vi "新剖面数据上传.vi"(11 "错误输入（无错误）":errorcluster) -> (15 "error out":errorcluster)   [LabVIEW 2016, in "数据传输系统-03.lvlib"]
uses:
  <vilib>/Utility/config.llb/Write Key (String).vi
  <vilib>/Utility/config.llb/Read Key (String).vi
  <vilib>/Utility/config.llb/NI_LVConfig.lvlib
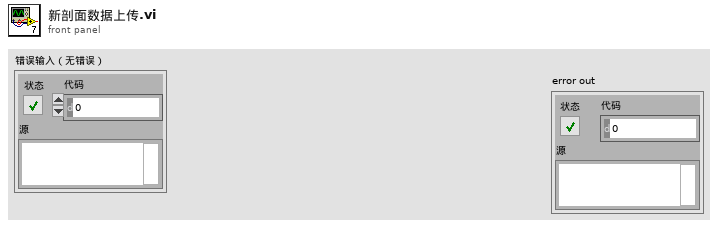
[diagram p1: front panel]
types:
  T1 = cluster{"setini":string, "sysini":string, "hechaini":string, "actualwrite":string, "actualread":string, "datasent":string, "反控命令信息队列":string, "反控与仪器交互":string}
  T2 = typedef "NI_LVConfig.lvlib/Config Data RefNum.ctl" = refnum<k1>
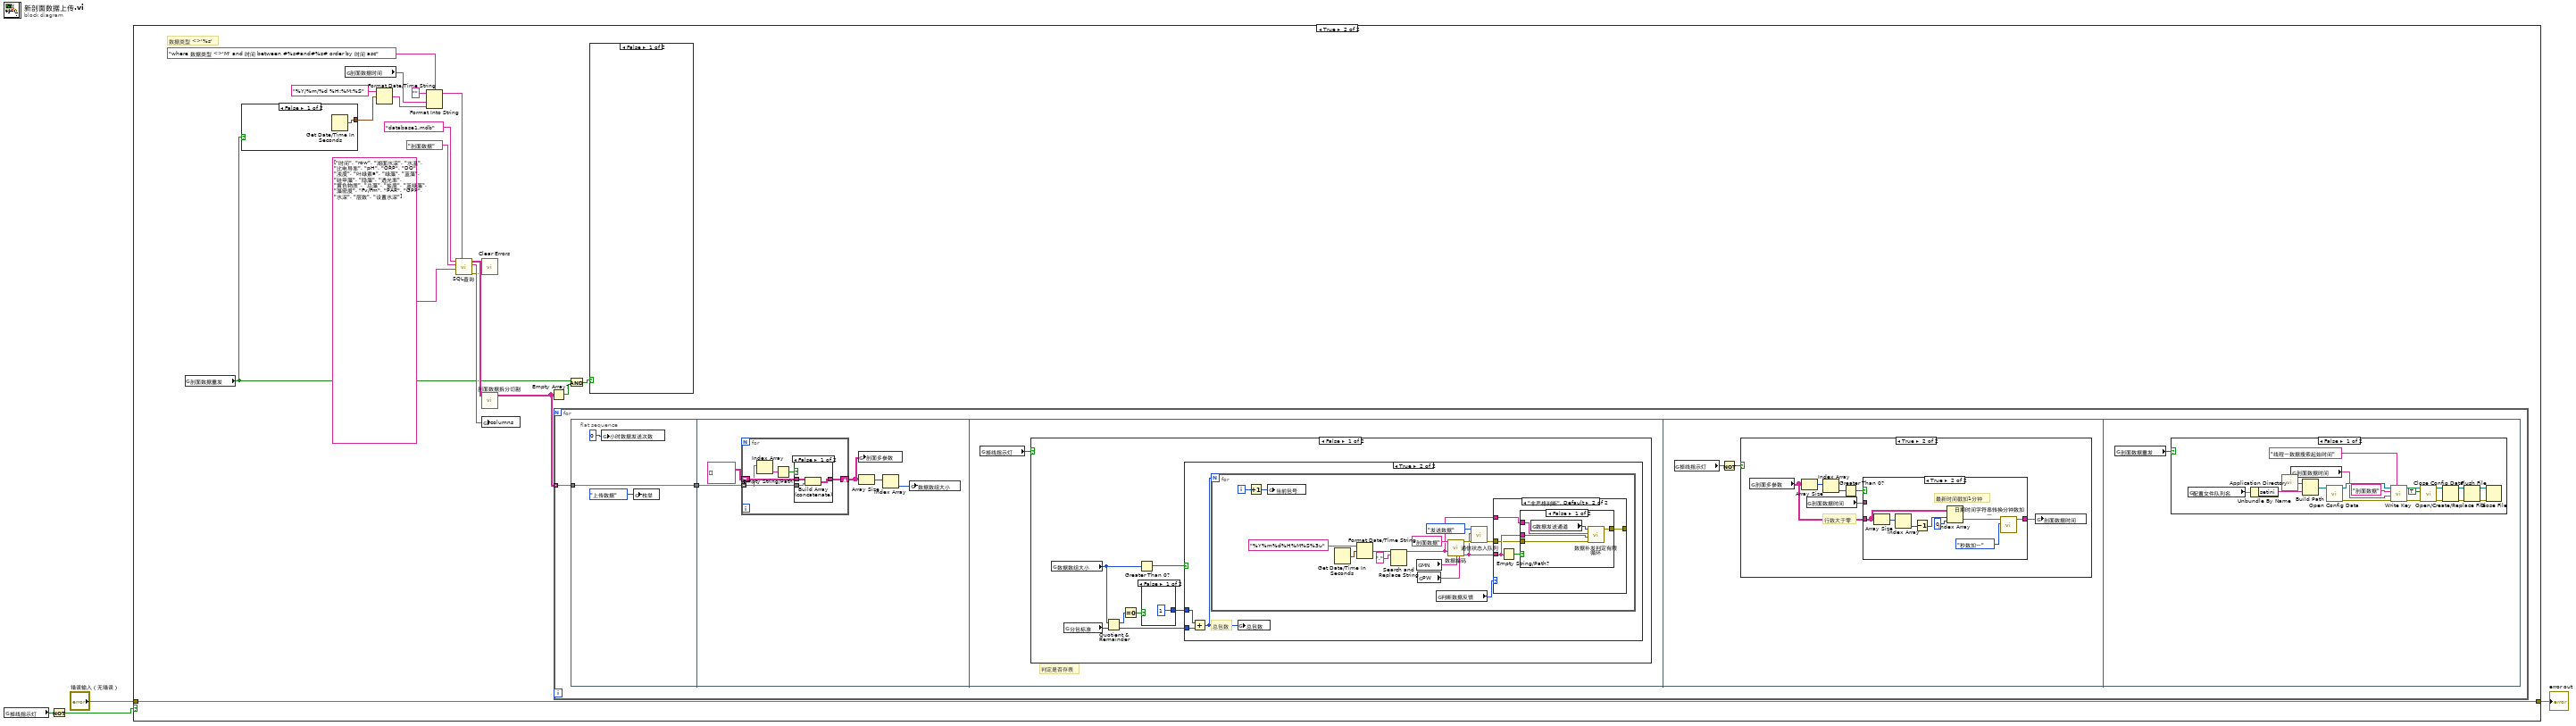
[diagram p0: block diagram]
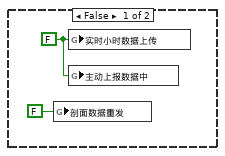
[diagram p2: hidden frame]
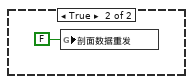
[diagram p3: hidden frame]
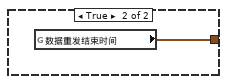
[diagram p4: hidden frame]
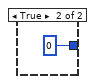
[diagram p6: hidden frame]
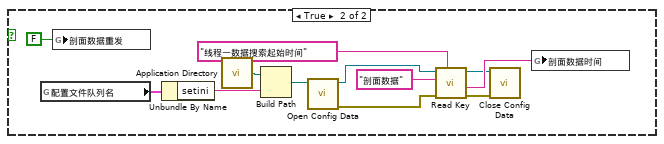
[diagram p13: hidden frame]
diagram:
  n1 = global read "全局 数据发送重叠.vi" "掉线指示灯"() -> (w4:bool)
  n2 = Not(x=w4) -> (.not. x?=w1:bool)
  n3 = case shown="True" w1 {
    tunnel: [_ w24] -> w3
    tunnel: "错误输入（无错误）" -> [_ w24]
    frame False {
      w6 = FALSE ("小时数据上传")
      n4 = global write "断电保存全局.vi" "剖面数据重发"(FALSE ("剖面数据重发")) -> ()
      n5 = global write "全局1.vi" "实时小时数据上传"(w6) -> ()
      n6 = global write "全局 数据发送重叠.vi" "主动上报数据中"(w6) -> ()
    }
    frame True {
      # "数据类型 <>'%s'"
      n7 = global read "断电保存全局.vi" "剖面数据重发"() -> (w8:bool)
      n8 = case shown="False" w8 {
        tunnel: [w26 w27] -> w11
        frame False {
          n9 = Get Date/Time In Seconds() -> (seconds since 1Jan1904=w26:timestamp)
        }
        frame True {
          n10 = global read "断电保存全局.vi" "数据重发结束时间"() -> (w27:timestamp)
        }
      }
      n11 = global read "全局 水样时间.vi" "剖面数据时间"() -> (w17:string)
      n12 = Format Date/Time String(time format string (%c)="%Y/%m/%d %H:%M:%S" ("时间格式字符串(%c)"), seconds (now)=w11) -> (date/time string=w16:string)  [unwired: 1 in]
      n13 = Format Into String(format string="where 数据类型 <>'M' and 时间 between #%s#and#%s# order by 时间 asc" ("condition"), initial string="" ("初始字符串"), w17, w16) -> (resulting string=w15:string)  [unwired: 1 in, 1 out]
      n14 = call "SQL查询.vi"("condition"=w15, "columns"=string[] ["时间", "row", "湖面水深", "水温", "比电导率", "pH", "ORP", "DO", "浊度", "叶绿素a", "绿藻", "蓝藻", "硅甲藻", "隐藻", "透光率", "黄色物质", "总藻", "盐度", "蓝绿藻", "藻密度", "Fv/Fm", "PAR", "GPP", "水深", "层数", "设置水深"], "table输入"="剖面数据", "database"="database1.mdb") -> ("error out"=w13:errorcluster, "columns输出"=w14:string[], "data"=w23:string[][])  [unwired: 4 in, 1 out]
      n15 = call <vilib>:"Clear Errors.vi"("error in (no error)"=w13) -> ()  [unwired: 5 in, 2 out]
      n16 = call "剖面数据拆分切割.vi"("剖面多参数输入"=w23) -> ("剖面多参数输出"=w10:string[][][])  [unwired: 10 in]
      n17 = global write "全局 所有参数.vi" "columns"(w14) -> ()
      n18 = Empty Array?(array=w10) -> (empty?=w7:bool)
      n19 = for {
        tunnel: w10 -> [w29] mode=indexing
        n20 = flat-sequence {
          tunnel: w29 -> [w32]
          tunnel: [w32] -> w28
          tunnel: w28 -> [w35]
          frame #0 {
            n21 = global write "全局 小时数据发送次数.vi" "小时数据发送次数"(0 ("小时数据发送次数")) -> ()
            n22 = global write "全局1.vi" "枚举"(enum16{"返回请求应答", "上传数据", "返回执行结果"}."上传数据" ("枚举")) -> ()
          }
          frame #1 {
            n23 = for {
              tunnel: w35 -> [w40] mode=indexing
              shift-right: [w41] -> w33
              shift-left: string[][] [] ("剖面多参数输入") -> [w42]
              n24 = Index Array(array=w40) -> (element=w39:string)  [unwired: 1 in]
              n25 = Empty String/Path?(string/path=w39) -> (empty?=w38:bool)
              n26 = case shown="False" w38 {
                tunnel: w42 -> [w45 w46]
                tunnel: w40 -> [w44 _]
                tunnel: [w43 w46] -> w41
                frame False {
                  n27 = Build Array (concatenate)(w45, w44) -> (w43:string[][])
                }
                frame True {
                }
              }
            }
            n28 = global write "全局 所有参数.vi" "剖面多参数"(w33) -> ()
            n29 = Array Size(array=w33) -> (size(s)=w36:i32[])
            n30 = Index Array(array=w36) -> (element=w37:i32)  [unwired: 1 in]
            n31 = global write "全局 数据数组大小.vi" "数据数组大小"(w37) -> ()
          }
          frame #2 {
            # "判定是否存表"
            n32 = global read "全局 数据发送重叠.vi" "掉线指示灯"() -> (w47:bool)
            n33 = case shown="False" w47 {
              frame False {
                n34 = global read "全局 数据数组大小.vi" "数据数组大小"() -> (w53:i32)
                n35 = global read "全局 数据数组大小.vi" "分包标准"() -> (w51:i32)
                n36 = Quotient & Remainder(x=w53, y=w51) -> (x-y*floor(x/y)=w50:i32, floor(x/y)=w52:i32)
                n37 = Equal To 0?(x=w50) -> (x = 0?=w49:bool)
                n38 = Greater Than 0?(x=w53) -> (x > 0?=w54:bool)
                n39 = case shown="False" w49 {
                  tunnel: [1 ("x") 0 ("x")] -> w48
                  frame False {
                  }
                  frame True {
                  }
                }
                n40 = case shown="True" w54 {
                  tunnel: w52 -> [_ w59]
                  tunnel: w48 -> [_ w57]
                  frame False {
                  }
                  frame True {
                    # "总包数"
                    n41 = Add(x=w57, y=w59) -> (x+y=w58:i32)
                    n42 = for {
                      N: w58 -> [_]
                      i -> [w67]
                      n43 = Increment(x=w67) -> (x+1=w66:i32)
                      n44 = global write "全局 数据数组大小.vi" "当前包号"(w66) -> ()
                      n45 = Get Date/Time In Seconds() -> (seconds since 1Jan1904=w72:timestamp)
                      n46 = Format Date/Time String(time format string (%c)="%Y%m%d%H%M%S%3u" ("时间格式字符串(%c)"), seconds (now)=w72) -> (date/time string=w71:string)  [unwired: 1 in]
                      n47 = Search and Replace String(input string=w71, search string="." ("搜索字符串")) -> (result string=w61:string)  [unwired: 6 in, 3 out]
                      n48 = global read "断电保存全局.vi" "MN"() -> (w64:string)
                      n49 = global read "断电保存全局.vi" "PW"() -> (w69:string)
                      n50 = global read "断电保存全局.vi" "判断数据反馈"() -> (w60:enum16{"非严格判断", "严格判断", "不判断"})
                      n51 = call "数据编码.vi"("table输入"="剖面数据" ("新元素/子数组"), "QN"=w61, "MN"=w64, "PW"=w69) -> ("错误常量"=w68:errorcluster, "通讯包字符串"=w62:string)  [unwired: 10 in]
                      n52 = call "通信状态入队列.vi"("错误输入（无错误）"=w68, "发送报文"=w62, "枚举"=enum16{"打开连接", "发送数据", "读取数据", "数据处理", "关闭连接"}."发送数据") -> ("错误输出"=w63:errorcluster)  [unwired: 8 in]
                      n53 = case shown="\"非严格判断\", Default" w60 {
                        tunnel: [_ w79] -> _
                        tunnel: w62 -> [_ w78]
                        tunnel: w61 -> [_ w77]
                        tunnel: w63 -> [_ w75]
                        frame "不判断" {
                        }
                        frame "非严格判断", Default {
                          n54 = Empty String/Path?(string/path=w78) -> (empty?=w76:bool)
                          n55 = case shown="False" w76 {
                            tunnel: [w84 _] -> w79
                            tunnel: w78 -> [w83 _]
                            tunnel: w77 -> [w81 _]
                            tunnel: w75 -> [w80 _]
                            frame False {
                              n56 = global read "断电保存全局.vi" "数据发送通道"() -> (w82:enum16{"TCP", "VISA"})
                              n57 = call "数据补发判定有限循环.vi"("错误输入（无错误）"=w80, "数据输入"=w83, "QN"=w81, "数据发送通道"=w82) -> ("error out"=w84:errorcluster)  [unwired: 7 in]
                            }
                            frame True {
                            }
                          }
                        }
                      }
                    }
                    n58 = global write "全局 数据数组大小.vi" "总包数"(w58) -> ()
                  }
                }
              }
              frame True {
              }
            }
          }
          frame #3 {
            n59 = global read "全局 数据发送重叠.vi" "掉线指示灯"() -> (w85:bool)
            n60 = Not(x=w85) -> (.not. x?=w86:bool)
            n61 = case shown="True" w86 {
              frame False {
              }
              frame True {
                # "行数大于零"
                n62 = global read "全局 所有参数.vi" "剖面多参数"() -> (w91:string[][])
                n63 = Array Size(array=w91) -> (size(s)=w88:i32[])
                n64 = global read "全局 水样时间.vi" "剖面数据时间"() -> (w92:string)
                n65 = Index Array(array=w88) -> (element=w89:i32)  [unwired: 1 in]
                n66 = Greater Than 0?(x=w89) -> (x > 0?=w90:bool)
                n67 = case shown="True" w90 {
                  tunnel: w91 -> [_ w98]
                  tunnel: [w93 w95] -> w87
                  tunnel: w92 -> [w93 _]
                  frame False {
                  }
                  frame True {
                    # "最新时间戳加1分钟"
                    n68 = Array Size(array=w98) -> (size(s)=w100:i32[])
                    n69 = Index Array(array=w100) -> (element=w99:i32)  [unwired: 1 in]
                    n70 = Decrement(x=w99) -> (x-1=w97:i32)
                    n71 = Index Array(array=w98, index (row)=w97, index (col)=0 ("禁用的索引 (列)")) -> (element=w101:string)
                    n72 = call "日期时间字符串转换分钟数加一.vi"("枚举"=enum16{"分钟数加一", "秒数加一", "小时数加一"}."秒数加一", "data[0]"=w101) -> ("日期/时间字符串"=w95:string)  [unwired: 9 in]
                  }
                }
                n73 = global write "全局 水样时间.vi" "剖面数据时间"(w87) -> ()
              }
            }
          }
          frame #4 {
            n74 = global read "断电保存全局.vi" "剖面数据重发"() -> (w102:bool)
            n75 = case shown="False" w102 {
              frame False {
                n76 = global read "全局1.vi" "配置文件队列名"() -> (w104:T1)
                n77 = Unbundle By Name(w104) -> ("setini"=w105:string)
                n78 = call <vilib>:"Application Directory.vi"() -> ("Application Directory"=w114:path)
                n79 = global read "全局 水样时间.vi" "剖面数据时间"() -> (w106:string)
                n80 = Build Path(base path=w114, name or relative path=w105) -> (appended path=w115:path)
                n81 = call <vilib>:"Open Config Data.vi"("configuration file path"=w115) -> ("error out"=w117:errorcluster, "refnum"=w116:T2)  [unwired: 8 in, 1 out]
                n82 = call-poly <vilib>:"Write Key.vi"("section"="线程一数据搜索起始时间", "error in (no error)"=w117, "value"=w106, "key"="剖面数据", "refnum"=w116) -> ("error out"=w119:errorcluster, "refnum out"=w118:T2)  [unwired: 4 in, 1 out]
                n83 = call <vilib>:"Close Config Data.vi"("error in (no error)"=w119, "write file if changed (T)"=TRUE, "refnum"=w118) -> ("error out"=w107:errorcluster, "file path"=w108:path)  [unwired: 7 in]
                n84 = Open/Create/Replace File(file path (use dialog)=w108, error in=w107) -> (refnum out=w110:refnum<file>, error out=w109:errorcluster)  [unwired: 4 in, 1 out]
                n85 = Flush File(refnum=w110, error in=w109) -> (refnum out=w111:refnum<file>, error out=w112:errorcluster)
                n86 = Close File(refnum=w111, error in=w112) -> ()  [unwired: 2 out]
              }
              frame True {
                n87 = global read "全局1.vi" "配置文件队列名"() -> (w121:T1)
                n88 = global write "断电保存全局.vi" "剖面数据重发"(FALSE ("剖面数据重发")) -> ()
                n89 = Unbundle By Name(w121) -> ("setini"=w129:string)
                n90 = call <vilib>:"Application Directory.vi"() -> ("Application Directory"=w128:path)
                n91 = Build Path(base path=w128, name or relative path=w129) -> (appended path=w130:path)
                n92 = call <vilib>:"Open Config Data.vi"("configuration file path"=w130) -> ("error out"=w125:errorcluster, "refnum"=w124:T2)  [unwired: 8 in, 1 out]
                n93 = call-poly <vilib>:"Read Key.vi"("section"="线程一数据搜索起始时间", "error in (no error)"=w125, "key"="剖面数据", "refnum"=w124) -> ("error out"=w127:errorcluster, "value"=w132:string, "refnum out"=w126:T2)  [unwired: 4 in, 1 out]
                n94 = call <vilib>:"Close Config Data.vi"("error in (no error)"=w127, "refnum"=w126) -> ()  [unwired: 8 in, 2 out]
                n95 = global write "全局 水样时间.vi" "剖面数据时间"(w132) -> ()
              }
            }
          }
        }
      }
      n96 = And(x=w8, y=w7) -> (x .and. y?=w9:bool)
      n97 = case shown="False" w9 {
        frame False {
        }
        frame True {
          n98 = global write "断电保存全局.vi" "剖面数据重发"(FALSE ("剖面数据重发")) -> ()
        }
      }
    }
  }
  "error out" <- w3
